vi "Read RAW Possition.vi"(0 "class data in":refnum<class "MB_ENGINE.lvclass">, 11 "error in (no error)":errorcluster) -> (4 "class data out":refnum<class "MB_ENGINE.lvclass">, 6 "RAW Possition":i32, 15 "error out":errorcluster)   [LabVIEW 2019, in "MB_ENGINE.lvclass"]
uses:
  MB_ENGINE.lvclass
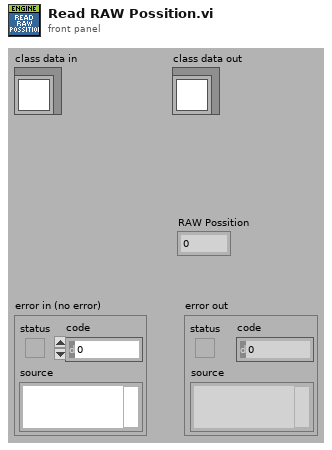
[diagram p1: front panel]
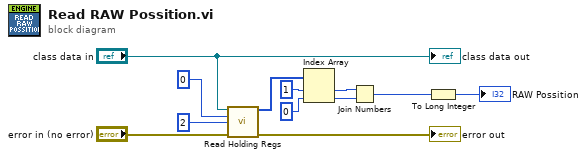
[diagram p0: block diagram]
diagram:
  n1 = call-dynamic "Read Holding Regs.vi"("reference in"="class data in", "starting address"=u16 0 ("y"), "number of inputs"=u16 2, "error in (no error)"="error in (no error)") -> ("register values"=w1:u16[], "error out"=→"error out":errorcluster)  [unwired: 10 in]
  n2 = Index Array(array=w1, index #1=1 ("index"), index #2=0 ("index")) -> (element #1=w5:u16, element #2=w4:u16)
  n3 = Join Numbers(hi=w5, lo=w4) -> ((hi.lo)=w9:u32)
  n4 = To Long Integer(number=w9) -> (32bit integer=→"RAW Possition":i32)
  "class data out" <- "class data in"
